vi "2dtilts_to_vector.vi"(1 "Array":cluster{dbl, dbl}[][](array[cluster])) -> (0 "Position":dbl[](array[numeric]))   [LabVIEW 2010]
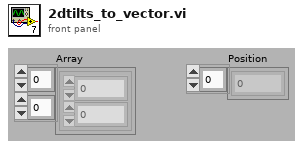
[diagram p1: front panel]
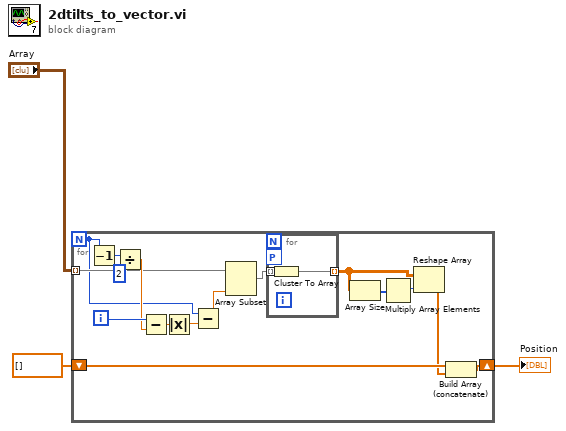
[diagram p0: block diagram]
diagram:
  n1 = for {
    N -> [w11]
    tunnel: "Array" -> [w14] mode=indexing
    shift-right: [w6] -> w1
    shift-left: dbl[] [] ("Position") -> [w5]
    i -> [w17]
    n2 = Decrement(x=w11) -> (x-1=w19:i32)
    n3 = Divide(x=w19, y=2) -> (x/y=w16:dbl)
    n4 = Subtract(x=w17, y=w16) -> (x-y=w13:dbl)
    n5 = Absolute Value(x=w13) -> (abs(x)=w12:dbl)
    n6 = Subtract(x=w11, y=w12) -> (x-y=w10:dbl)
    n7 = Array Subset(array=w14, length=w10) -> (w15:cluster{dbl, dbl}[])  [unwired: 1 in]
    n8 = for {
      tunnel: w15 -> [w21] mode=indexing
      tunnel: [w20] -> w7 mode=indexing
      workers-P: _ -> [_]
      n9 = Cluster To Array(cluster=w21) -> (array=w20:dbl[])
    }
    n10 = Array Size(array=w7) -> (size(s)=w8:i32[])
    n11 = Multiply Array Elements(1:w8) -> (0:w9:i32)
    n12 = Reshape Array(w7, w9) -> (w4:dbl[])
    n13 = Build Array (concatenate)(w5, w4) -> (w6:dbl[])
  }
  "Position" <- w1
